vi "dimDirxy.vi"(8 "Barrido X":bool, 10 "nY":i32, 11 "nX":i32) -> (2 "nXY":i32[](array[numeric]))   [LabVIEW 2018]
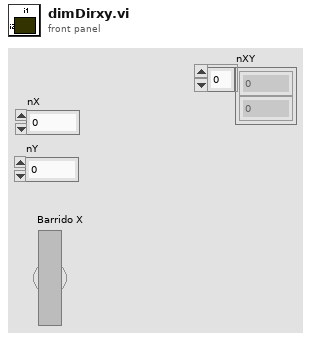
[diagram p1: front panel]
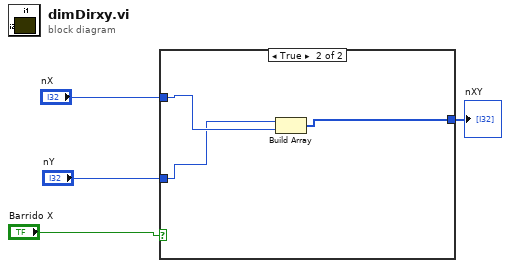
[diagram p0: block diagram]
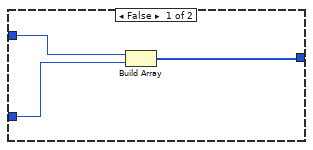
[diagram p2: hidden frame]
diagram:
  n1 = case shown="True" "Barrido X" {
    tunnel: "nX" -> [w7 w10]
    tunnel: "nY" -> [w6 w9]
    tunnel: [w5 w8] -> w1
    frame False {
      n2 = Build Array(w7, w6) -> (w5:i32[])
    }
    frame True {
      n3 = Build Array(w9, w10) -> (w8:i32[])
    }
  }
  "nXY" <- w1
